vi "Read QDEvent Logfile.vi"(8 "Error In":errorcluster, 10 "Quench Event Logfile":path, 11 "KIT-QA in":refnum<class "KIT-QA.lvclass">) -> (0 "Error Out":errorcluster, 3 "KIT-QA out":refnum<class "KIT-QA.lvclass">)   [LabVIEW 2015, in "KIT-QA.lvlib" / "KIT-QA.lvclass"]
uses:
  KIT-QA.lvclass
  KIT-QA.lvclass/KIT-QA.ctl
  <vilib>/ActorFramework/Actor/Actor.lvclass/Actor.ctl
  <vilib>/ActorFramework/Message Enqueuer/Message Enqueuer.lvclass/Message Enqueuer.ctl
  <vilib>/ActorFramework/Message Enqueuer/Init from Existing Queue.vi
  <vilib>/ActorFramework/Message Enqueuer/Enqueue.vi
  <vilib>/ActorFramework/Message Priority Queue/Priority Enqueue.vi
  <vilib>/ActorFramework/Message Enqueuer/Message Enqueuer.lvclass
  KIT-QA Messages/Read QD Raw Data Msg/Read QD Raw Data Msg.lvclass
  <vilib>/ActorFramework/Actor/Actor.lvclass
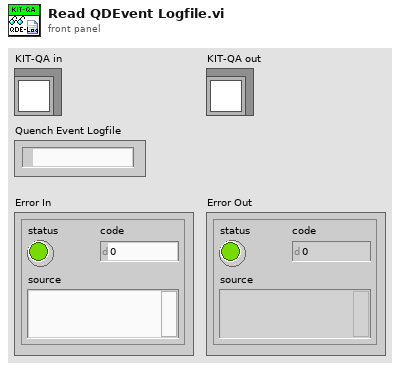
[diagram p1: front panel]
types:
  T1 = enum16{"open", "replace", "create", "open or create", "replace or create", "replace or create with confirmation"}
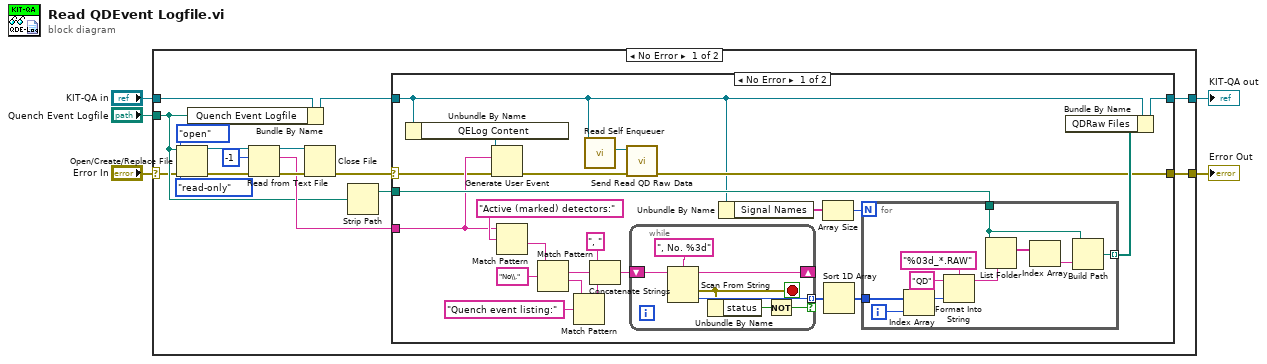
[diagram p0: block diagram]
diagram:
  n1 = case shown="No Error" "Error In" {
    selector: "Error In" -> [w11 w65]
    tunnel: [w9 w65] -> w4
    tunnel: [w8 w64] -> w2
    tunnel: "KIT-QA in" -> [w7 w64]
    tunnel: "Quench Event Logfile" -> [w12 _]
    frame No Error {
      n2 = Open/Create/Replace File(file path (use dialog)=w12, error in=w11, operation (0:open)=T1."open", access (0:read/write)=enum16{"read/write", "read-only", "write-only"}."read-only") -> (refnum out=w19:refnum<file>, error out=w18:errorcluster)  [unwired: 2 in, 1 out]
      n3 = Bundle By Name(cluster=w7, "Quench Event Logfile"=w12) -> (w6:refnum<class "KIT-QA.lvclass">)
      n4 = Read from Text File(file (use dialog)=w19, count=-1, error in=w18) -> (refnum out=w16:refnum<file>, text=w14:string, error out=w17:errorcluster)  [unwired: 1 in, 1 out]
      n5 = Close File(refnum=w16, error in=w17) -> (error out=w10:errorcluster)  [unwired: 1 out]
      n6 = Strip Path(path=w12) -> (stripped path=w13:path)  [unwired: 1 out]
      n7 = case shown="No Error" w10 {
        selector: w10 -> [w31 w63]
        tunnel: w14 -> [w32 _]
        tunnel: w13 -> [w35 _]
        tunnel: [w26 w63] -> w9
        tunnel: [w30 w62] -> w8
        tunnel: w6 -> [w24 w62]
        frame No Error {
          n8 = Unbundle By Name(w24) -> ("QELog Content"=w33:refnum<user-event>)
          n9 = Generate User Event(user event=w33, event data cluster=w32, error in=w31) -> (error out=w27:errorcluster)  [unwired: 1 in, 1 out]
          n10 = Match Pattern(string=w32, regular expression="Active (marked) detectors:") -> (after substring=w43:string)  [unwired: 1 in, 3 out]
          n11 = Match Pattern(string=w43, regular expression="No\\.") -> (match substring=w41:string, after substring=w40:string)  [unwired: 1 in, 2 out]
          n12 = Match Pattern(string=w40, regular expression="Quench event listing:") -> (before substring=w38:string)  [unwired: 1 in, 3 out]
          n13 = call <vilib>:"Read Self Enqueuer.vi"("Actor"=w24) -> ("Self Enqueuer"=w28:refnum<class "Message Enqueuer.lvclass">)  [unwired: 10 in]
          n14 = Concatenate Strings(", " ("string"), w41, w38) -> (w37:string)
          n15 = call "Send Read QD Raw Data.vi"("error in (no error)"=w27, "Message Enqueuer"=w28) -> ("error out"=w26:errorcluster)  [unwired: 8 in, 1 out]
          n16 = while {
            shift-right: [w60] -> _
            shift-left: w37 -> [w61]
            tunnel: [w58] -> w34 mode=indexing if=w56
            stop <- w57 stop-if-true
            n17 = Scan From String(format string=", No. %3d", input string=w61) -> (remaining string=w60:string, error out=w57:errorcluster, output 1=w58:i32)  [unwired: 3 in, 1 out]
            n18 = Unbundle By Name(w57) -> ("status"=w55:bool)
            n19 = Not(x=w55) -> (.not. x?=w56:bool)
          }
          n20 = Unbundle By Name(w24) -> ("Signal Names"=w23:string[])
          n21 = Array Size(array=w23) -> (size(s)=w22:i32)
          n22 = Sort 1D Array(array=w34) -> (sorted array=w25:i32[])
          n23 = for {
            N: w22 -> [_]
            tunnel: w35 -> [w50]
            tunnel: w25 -> [w48]
            tunnel: [w47] -> w29 mode=indexing
            i -> [w45]
            n24 = Index Array(array=w48, index=w45) -> (element=w46:i32)
            n25 = Format Into String(format string="%03d_*.RAW", initial string="QD" ("regular expression"), w46) -> (resulting string=w52:string)  [unwired: 1 in, 1 out]
            n26 = List Folder(path=w50, pattern=w52) -> (filenames=w51:string[])  [unwired: 2 in, 3 out]
            n27 = Index Array(array=w51) -> (element=w49:string)  [unwired: 1 in]
            n28 = Build Path(base path=w50, name or relative path=w49) -> (appended path=w47:path)
          }
          n29 = Bundle By Name(cluster=w24, "QDRaw Files"=w29) -> (w30:refnum<class "KIT-QA.lvclass">)
        }
        frame Error {
        }
      }
    }
    frame Error {
    }
  }
  "Error Out" <- w4
  "KIT-QA out" <- w2
